vi "2 VI Template (Without Error Terminals).vi"(1 "Input 2":string, 2 "Input 1":string) -> (0 "Output":string)   [LabVIEW 2021]
doc: "<add documentation here>"
panel:
  # "Development\nControls or indicators that are useful for development or testing, but which are not outputs of the VI."
  # "Input\nInputs to the VI"
  # "Output\nOutputs of the VI"
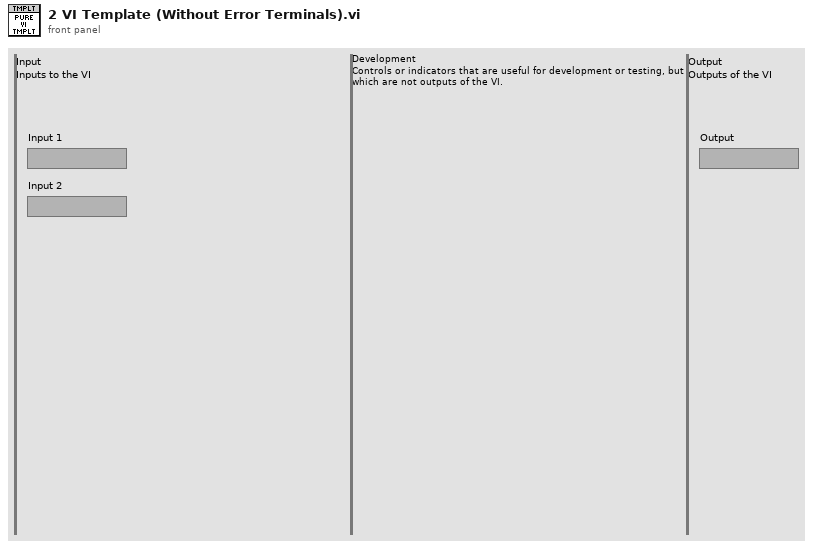
[diagram p1: front panel]
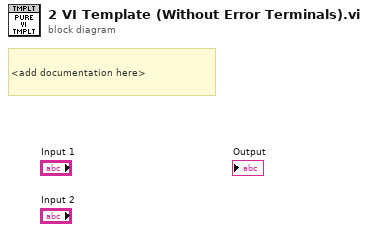
[diagram p0: block diagram]
diagram:
  # "<add documentation here>"
